vi "Periodic Tasks.vi"(8 "error in":errorcluster) -> ()   [LabVIEW 2025]
doc: "This VI runs in parallel to other tasks. It can contain as many user-defined periodic loops as you need. These can carry out PID or other sorts of timed response."
uses:
  GeneralPurpose/AllianceColorGlobal.vi
  <vilib>/Rock Robotics/Network Tables/NT Write String.vi
  <vilib>/Rock Robotics/Network Tables/NT Read String.vi
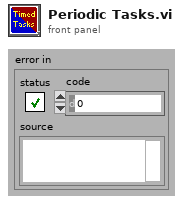
[diagram p1: front panel]
types:
  T1 = typedef "WPI_DriverStationAllianceInfo.ctl" = enum16{"Red", "Blue", "Invalid"}
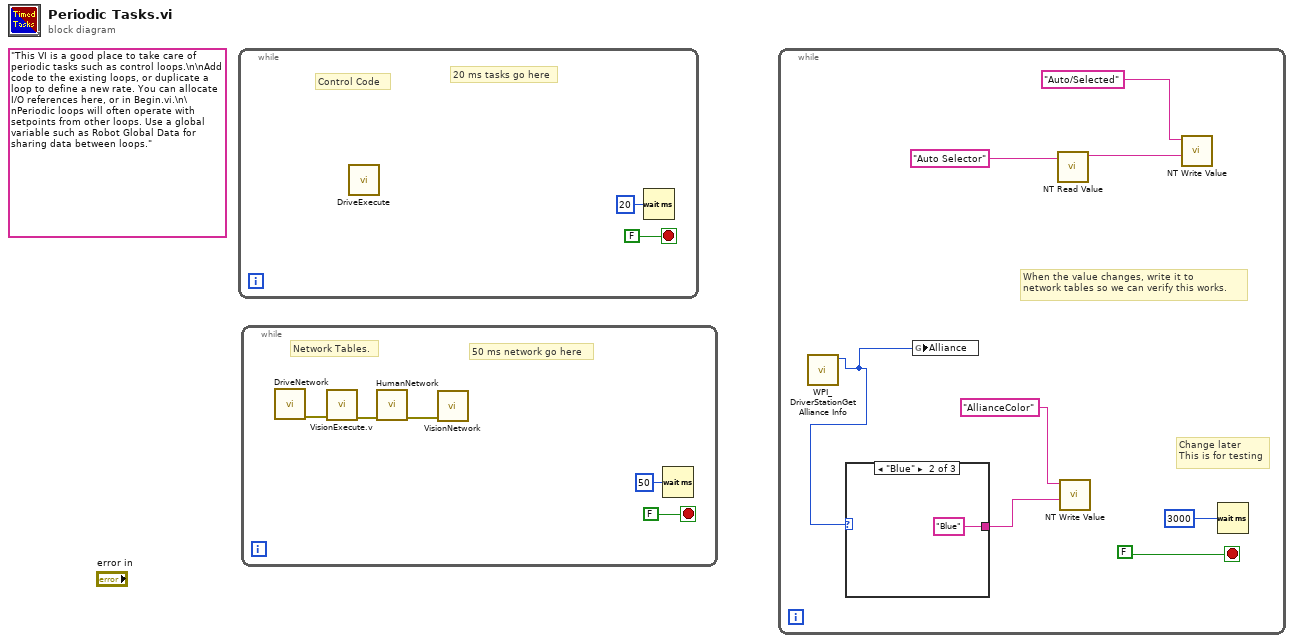
[diagram p0: block diagram]
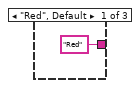
[diagram p2: hidden frame]
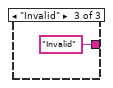
[diagram p3: hidden frame]
diagram:
  (unwired) "This VI is a good place to take care of periodic tasks such as control loops.\n\nAdd code to the existing loops, or duplicate a loop to define a new rate. You can allocate I/O references here, or in Begin.vi.\n\nPeriodic loops will often operate with setpoints from other loops. Use a global variable such as Robot Global Data for sharing data between loops."
  n1 = while {
    stop <- FALSE stop-if-true
    # "Control Code"
    # "20 ms tasks go here"
    n2 = call "DriveExecute.vi"() -> ()  [unwired: 11 in, 1 out]
    n3 = Wait (ms)(milliseconds to wait=u32 20) -> ()  [unwired: 1 out]
  }
  n4 = while {
    stop <- FALSE stop-if-true
    # "Network Tables."
    # "50 ms network go here"
    n5 = call "DriveNetwork.vi"() -> ("error out"=w4:errorcluster)  [unwired: 11 in]
    n6 = call "VisionExecute.v.vi"("error in (no error)"=w4) -> ("error out"=w3:errorcluster)  [unwired: 10 in]
    n7 = call "HumanNetwork.vi"("error in (no error)"=w3) -> ("error out"=w5:errorcluster)  [unwired: 10 in]
    n8 = call "VisionNetwork.vi"("error in (no error)"=w5) -> ()  [unwired: 10 in, 1 out]
    n9 = Wait (ms)(milliseconds to wait=u32 50) -> ()  [unwired: 1 out]
  }
  n10 = while {
    stop <- FALSE stop-if-true
    # "When the value changes, write it to \nnetwork tables so we can verify this works."
    # "Change later\nThis is for testing"
    n11 = call <vilib>:"WPI_DriverStationGet Alliance Info.vi"() -> ("Alliance"=w13:T1)  [unwired: 6 in, 5 out]
    n12 = case shown="\"Blue\"" w13 {
      tunnel: ["Red" "Blue" "Invalid"] -> w12
      frame "Red", Default {
      }
      frame "Blue" {
      }
      frame "Invalid" {
      }
    }
    n13 = global write "AllianceColorGlobal.vi" "Alliance"(w13) -> ()
    n14 = call-poly <vilib>:"NT Read Value.vi"("name"="Auto Selector" ("Name")) -> ("value"=w8:string)  [unwired: 8 in, 2 out]
    n15 = call-poly <vilib>:"NT Write Value.vi"("value"=w12, "name"="AllianceColor") -> ()  [unwired: 9 in, 1 out]
    n16 = call-poly <vilib>:"NT Write Value.vi"("value"=w8, "name"="Auto/Selected") -> ()  [unwired: 9 in, 1 out]
    n17 = Wait (ms)(milliseconds to wait=u32 3000) -> ()  [unwired: 1 out]
  }
